vi "Check Vehicle Exit.vi"(8 "error in (no error)":errorcluster, 11 "Vehicle Position Simulation in":refnum<class "Vehicle Position Simulation.lvclass">) -> (0 "error out":errorcluster, 3 "Vehicle Position Simulation out":refnum<class "Vehicle Position Simulation.lvclass">)   [LabVIEW 2019, in "Vehicle Position Simulation.lvlib" / "Vehicle Position Simulation.lvclass"]
uses:
  Vehicle Position Simulation.lvclass
  Vehicle Position Simulation.lvclass/Vehicle Position Simulation.ctl
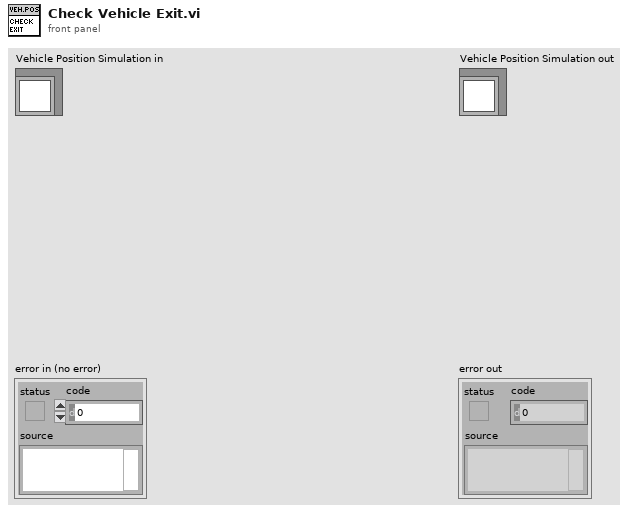
[diagram p1: front panel]
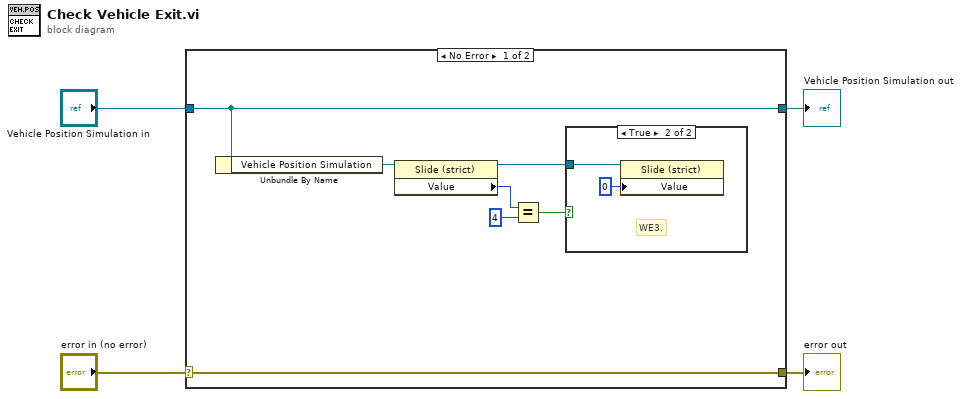
[diagram p0: block diagram]
diagram:
  n1 = case shown="No Error" "error in (no error)" {
    selector: "error in (no error)" -> [w11 w15]
    tunnel: [w11 w15] -> w3
    tunnel: [w10 w14] -> w1
    tunnel: "Vehicle Position Simulation in" -> [w10 w14]
    frame No Error {
      n2 = Unbundle By Name(w10) -> ("Vehicle Position Simulation"=w9:refnum<vi>)
      n3 = property class="Slide (strict)"(reference=w9) -> (reference out=w5:refnum<vi>, "Value"=w8:u32)  [unwired: 1 in, 1 out]
      n4 = Equal?(x=w8, y=u32 4) -> (x = y?=w6:bool)
      n5 = case shown="True" w6 {
        tunnel: w5 -> [_ w13]
        frame False {
        }
        frame True {
          # "WE3."
          n6 = property class="Slide (strict)"(reference=w13, "Value"=u32 0) -> ()  [unwired: 1 in, 2 out]
        }
      }
    }
    frame Error {
    }
  }
  "error out" <- w3
  "Vehicle Position Simulation out" <- w1
